vi "SimpleGit-Pull.vi"(11 "path":path) -> ()   [LabVIEW 2017]
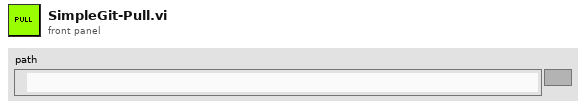
[diagram p1: front panel]
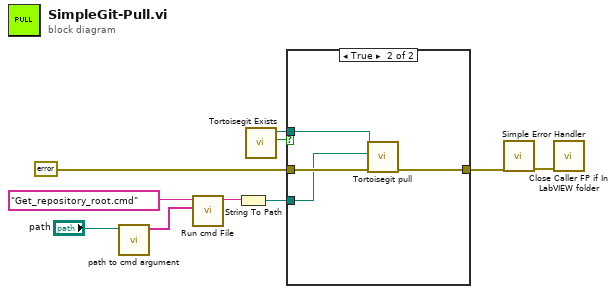
[diagram p0: block diagram]
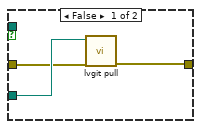
[diagram p2: hidden frame]
diagram:
  n1 = call "path to cmd argument.vi"("path"="path") -> ("Array"=w5:string[])  [unwired: 10 in]
  n2 = call "Run cmd File.vi"("args"=w5, "name or relative path"="Get_repository_root.cmd") -> ("standard output"=w2:string)  [unwired: 7 in, 2 out]
  n3 = String To Path(string=w2) -> (path=w1:path)
  n4 = call "Tortoisegit Exists.vi"() -> ("file or folder exists?"=w9:bool, "TortoiseGitProc.exe"=w8:path)  [unwired: 10 in]
  n5 = case shown="True" w9 {
    tunnel: errorcluster {"status"=FALSE, "code"=0, "source"=""} ("error out") -> [w12 w17]
    tunnel: w8 -> [_ w15]
    tunnel: w1 -> [w13 w16]
    tunnel: [w11 w14] -> w7
    frame False {
      n6 = call "lvgit pull.vi"("error in"=w12, "path"=w13) -> ("error out"=w11:errorcluster)  [unwired: 9 in]
    }
    frame True {
      n7 = call "Tortoisegit pull.vi"("error in (no error)"=w17, "path"=w16, "TortoiseGitProc.exe"=w15) -> ("error out"=w14:errorcluster)  [unwired: 8 in]
    }
  }
  n8 = call <vilib>:"Simple Error Handler.vi"("error in (no error)"=w7) -> ("error out"=w10:errorcluster)  [unwired: 4 in, 4 out]
  n9 = call "Close Caller FP if In LabVIEW folder.vi"("error in (no error)"=w10) -> ()  [unwired: 10 in, 1 out]
